vi "FL defuzzify output variables.vi"(7 "max num consequent membership fcns":i32, 9 "output membership factors (u)":dbl[][](array[numeric]), 11 "fuzzy system in":T1={"input variables"=[], "output variables"=[], "rules"=[], "defuzzification method"=0, "description"="\r\n", "user MF interpolating polynomials"=[]} {"user MF interpolating polynomials"."coa_x(y) coeff" format="%.4g"; "user MF interpolating polynomials"."Area(y) coeff" format="%.4g"; "user MF interpolating polynomials"."X(y) coeff" format="%.4g"; "user MF interpolating polynomials"."Y(x) coeff" format="%.4g"; "user MF interpolating polynomials"."Y" format="%.4g"; "user MF interpolating polynomials"."X" format="%.4g"; "defuzzification method" items=["Center of Area", "Modified Center of Area", "Center of Sums", "Center of Maximum", "Mean of Maximum"]; "rules"."consequents"."Var Index" min=0; "rules"."consequents"."Cond" items=["=", "!="]; "rules"."consequents"."MF Index" min=0; "rules"."antecedents"."Var Index" min=0; "rules"."antecedents"."Cond" items=["=", "!="]; "rules"."antecedents"."MF Index" min=0; "rules"."consequent implication" items=["Minimum", "Product"]; "rules"."antecedent connective" items=["AND (Minimum)", "AND (Product)", "OR (Maximum)", "OR (Probabilistic)"]; "output variables"."MFs"."shape" items=["Triangle", "Trapezoid", "Singleton", "Sigmoid", "Gaussian", "User-Defined"]; "input variables"."MFs"."shape" items=["Triangle", "Trapezoid", "Singleton", "Sigmoid", "Gaussian", "User-Defined"]}) -> (1 "output membership factors (u)":dbl[][](array[numeric]), 2 "output variables":dbl[](array[numeric])=[2.4048035734913955], 3 "fuzzy system out":T1 {"user MF interpolating polynomials"."coa_x(y) coeff" format="%.4g"; "user MF interpolating polynomials"."Area(y) coeff" format="%.4g"; "user MF interpolating polynomials"."X(y) coeff" format="%.4g"; "user MF interpolating polynomials"."Y(x) coeff" format="%.4g"; "user MF interpolating polynomials"."Y" format="%.4g"; "user MF interpolating polynomials"."X" format="%.4g"; "defuzzification method" items=["Center of Area", "Modified Center of Area", "Center of Sums", "Center of Maximum", "Mean of Maximum"]; "rules"."consequents"."Var Index" min=0; "rules"."consequents"."Cond" items=["=", "!="]; "rules"."consequents"."MF Index" min=0; "rules"."antecedents"."Var Index" min=0; "rules"."antecedents"."Cond" items=["=", "!="]; "rules"."antecedents"."MF Index" min=0; "rules"."consequent implication" items=["Minimum", "Product"]; "rules"."antecedent connective" items=["AND (Minimum)", "AND (Product)", "OR (Maximum)", "OR (Probabilistic)"]; "output variables"."MFs"."shape" items=["Triangle", "Trapezoid", "Singleton", "Sigmoid", "Gaussian", "User-Defined"]; "input variables"."MFs"."shape" items=["Triangle", "Trapezoid", "Singleton", "Sigmoid", "Gaussian", "User-Defined"]})   [LabVIEW 2020, in "NI_Fuzzy_Logic_API.lvlib"]
uses:
  <vilib>/addons/Fuzzy Logic/NI_Fuzzy_Logic_API.lvlib
  <vilib>/addons/Fuzzy Logic/TypeDefs/FL System.ctl
  <vilib>/addons/Fuzzy Logic/TypeDefs/FL Variable.ctl
  <vilib>/addons/Fuzzy Logic/TypeDefs/FL Membership Function.ctl
  <vilib>/addons/Fuzzy Logic/TypeDefs/FL Membership Function Shape.ctl
  <vilib>/addons/Fuzzy Logic/TypeDefs/FL Rule.ctl
  <vilib>/addons/Fuzzy Logic/TypeDefs/FL Antecedent.ctl
  <vilib>/addons/Fuzzy Logic/TypeDefs/FL Modifier.ctl
  <vilib>/addons/Fuzzy Logic/TypeDefs/FL Antecedent Connective.ctl
  <vilib>/addons/Fuzzy Logic/TypeDefs/FL Consequent.ctl
  <vilib>/addons/Fuzzy Logic/TypeDefs/FL Consequent Implication.ctl
  <vilib>/addons/Fuzzy Logic/TypeDefs/FL Defuzzification.ctl
  <vilib>/addons/Fuzzy Logic/TypeDefs/FL Interpolating polynomials.ctl
  <vilib>/Analysis/1siggen.llb/Ramp Pattern by Samples.vi
  <vilib>/Analysis/8numeric.llb/1D Numeric Integration.vi
  <vilib>/Analysis/NI_AALPro.lvlib
  <vilib>/Analysis/NI_AALBase.lvlib
panel:
  # "IF"
  # "THEN"
  # "IF"
  # "THEN"
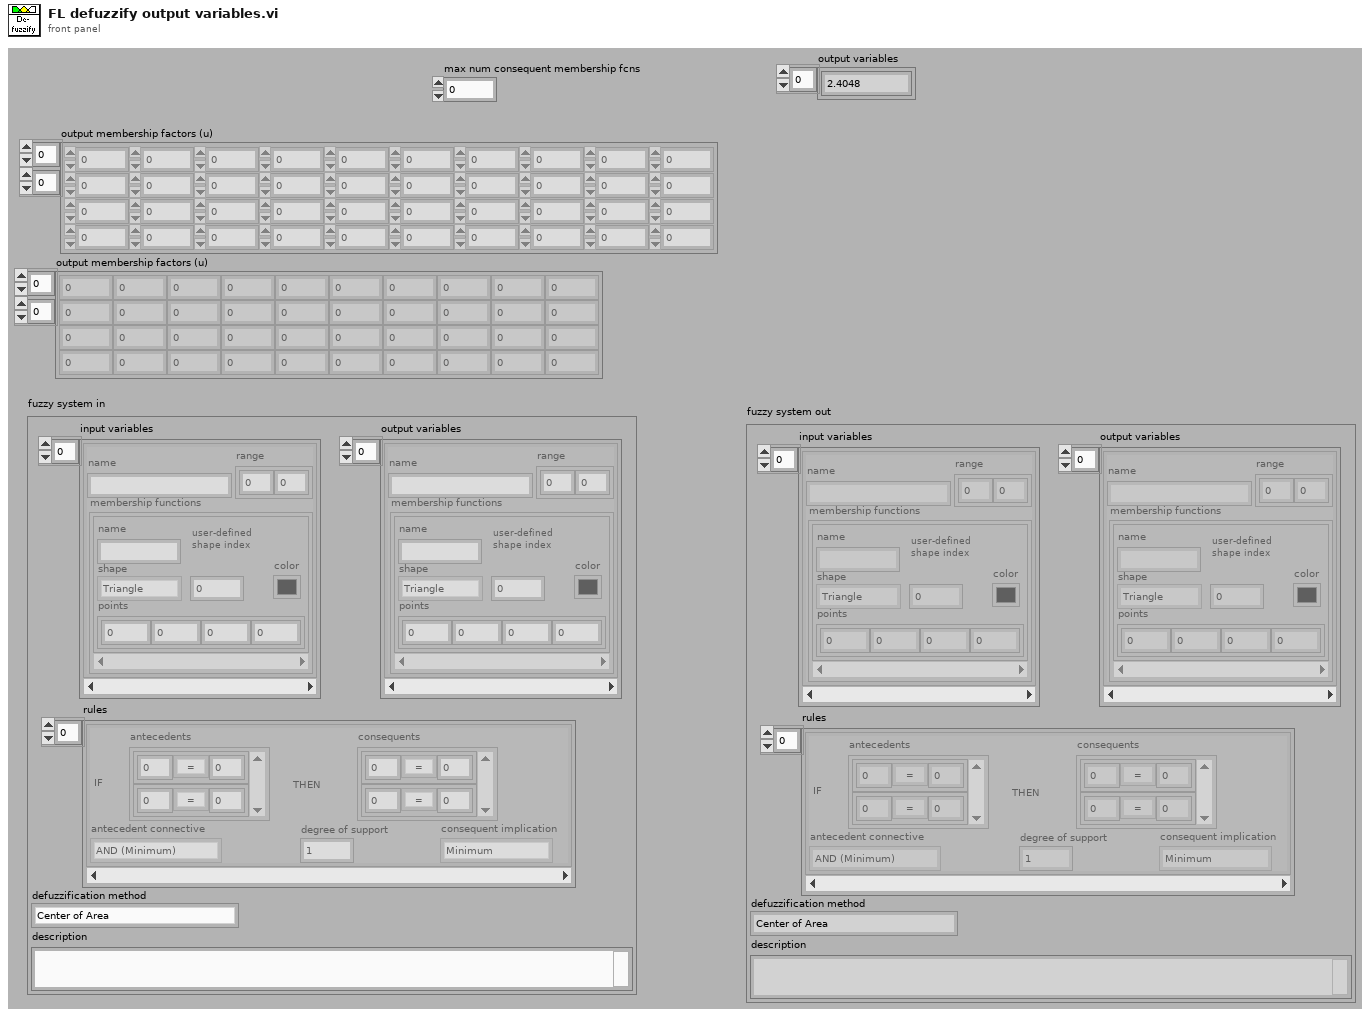
[diagram p1: front panel]
types:
  T1 = typedef "NI_Fuzzy_Logic_API.lvlib/FL System.ctl" = cluster{"input variables":T2[], "output variables":T2[], "rules":T5[], "defuzzification method":T11, "description":string, "user MF interpolating polynomials":T12[]}
  T2 = typedef "NI_Fuzzy_Logic_API.lvlib/FL Variable.ctl" = cluster{"name":string, "range":dbl[], "MFs":T3[]}
  T3 = typedef "NI_Fuzzy_Logic_API.lvlib/FL Membership Function.ctl" = cluster{"name":string, "shape":T4, "points":dbl[], "color":u32, "user-defined shape index":i32}
  T4 = typedef "NI_Fuzzy_Logic_API.lvlib/FL Membership Function Shape.ctl" = u16
  T5 = typedef "NI_Fuzzy_Logic_API.lvlib/FL Rule.ctl" = cluster{"antecedents":T6[], "antecedent connective":T8, "consequents":T9[], "consequent implication":T10, "degree of support":dbl}
  T6 = typedef "NI_Fuzzy_Logic_API.lvlib/FL Antecedent.ctl" = cluster{"Var Index":i32, "MF Index":i32, "Cond":T7}
  T7 = typedef "NI_Fuzzy_Logic_API.lvlib/FL Modifier.ctl" = u16
  T8 = typedef "NI_Fuzzy_Logic_API.lvlib/FL Antecedent Connective.ctl" = u16
  T9 = typedef "NI_Fuzzy_Logic_API.lvlib/FL Consequent.ctl" = cluster{"Var Index":i32, "MF Index":i32, "Cond":T7}
  T10 = typedef "NI_Fuzzy_Logic_API.lvlib/FL Consequent Implication.ctl" = u16
  T11 = typedef "NI_Fuzzy_Logic_API.lvlib/FL Defuzzification.ctl" = u16
  T12 = typedef "NI_Fuzzy_Logic_API.lvlib/FL Interpolating polynomials.ctl" = cluster{"X":dbl[], "Y":dbl[], "Y(x) coeff":dbl[][], "X(y) coeff":dbl[][], "Area(y) coeff":dbl[][], "coa_x(y) coeff":dbl[][]}
  T13 = enum32{"Trapezoidal Rule", "Simpson's Rule", "Simpson's 3/8 Rule", "Bode Rule"}
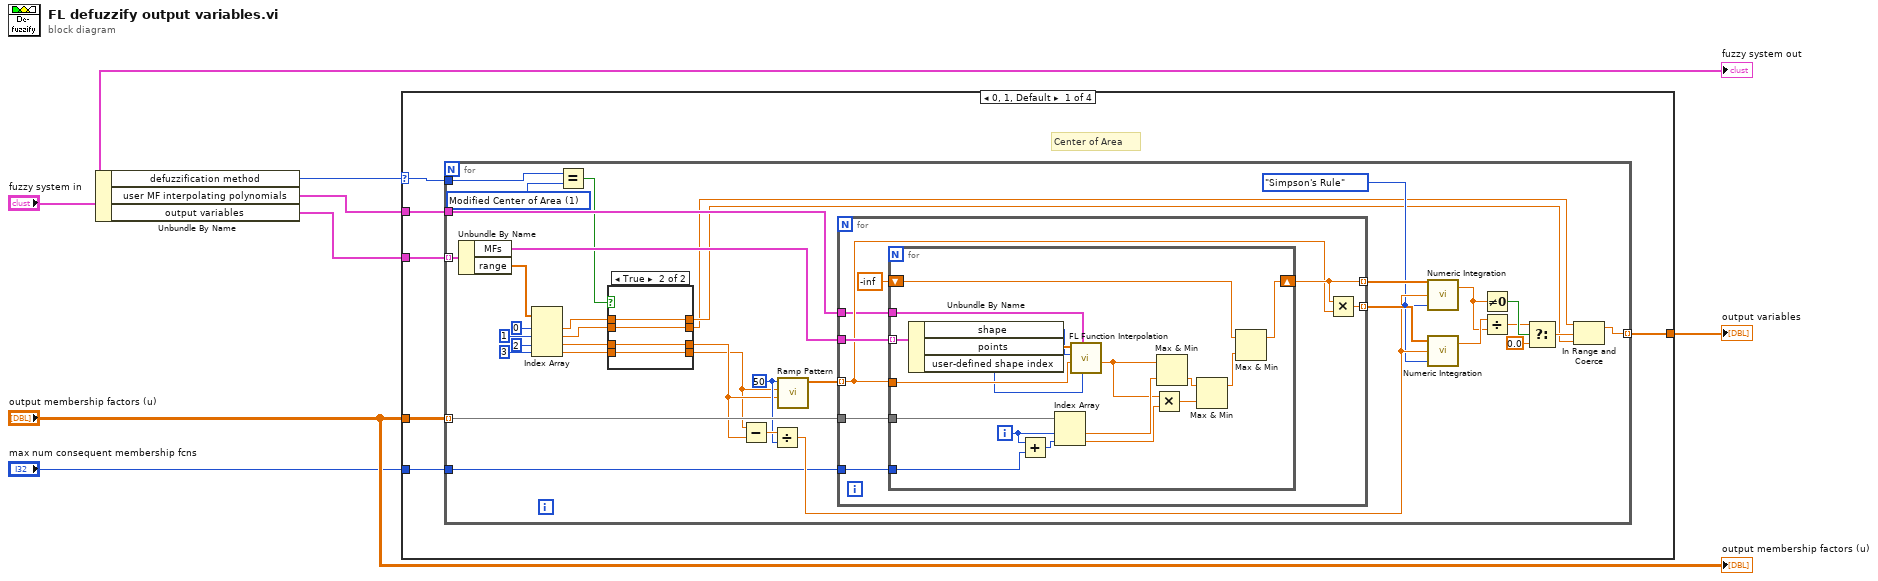
[diagram p0: block diagram]
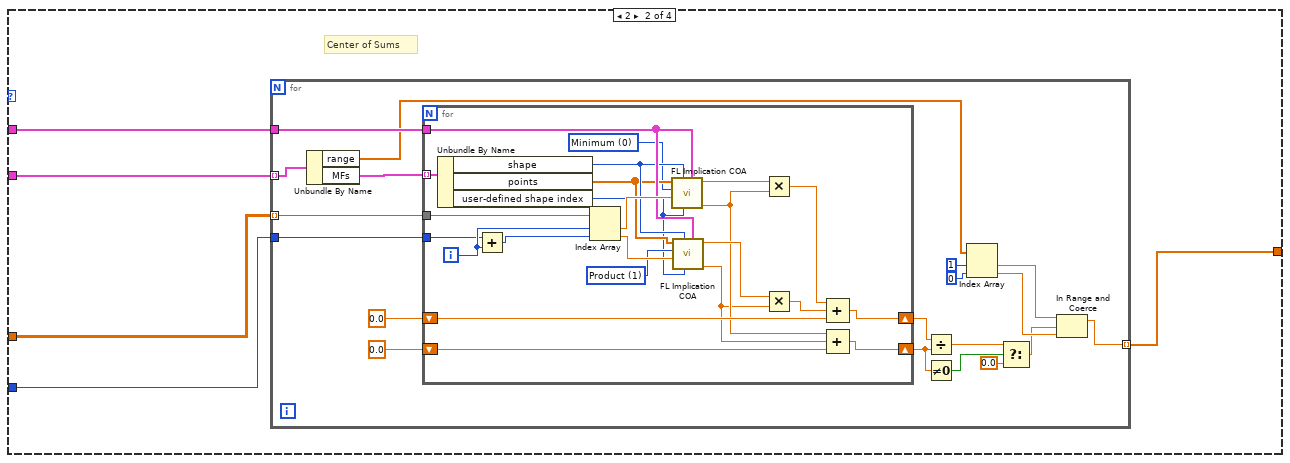
[diagram p3: hidden frame]
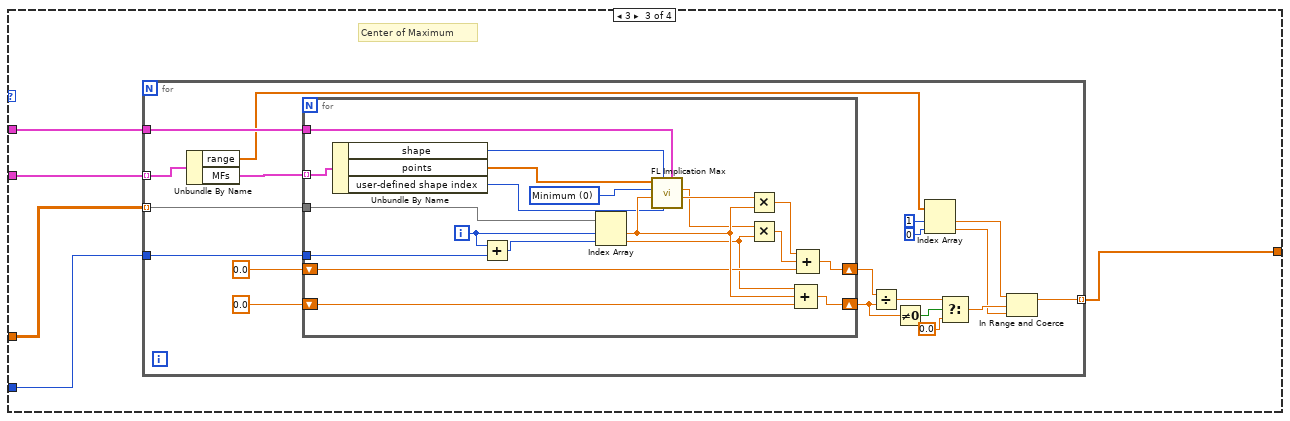
[diagram p4: hidden frame]
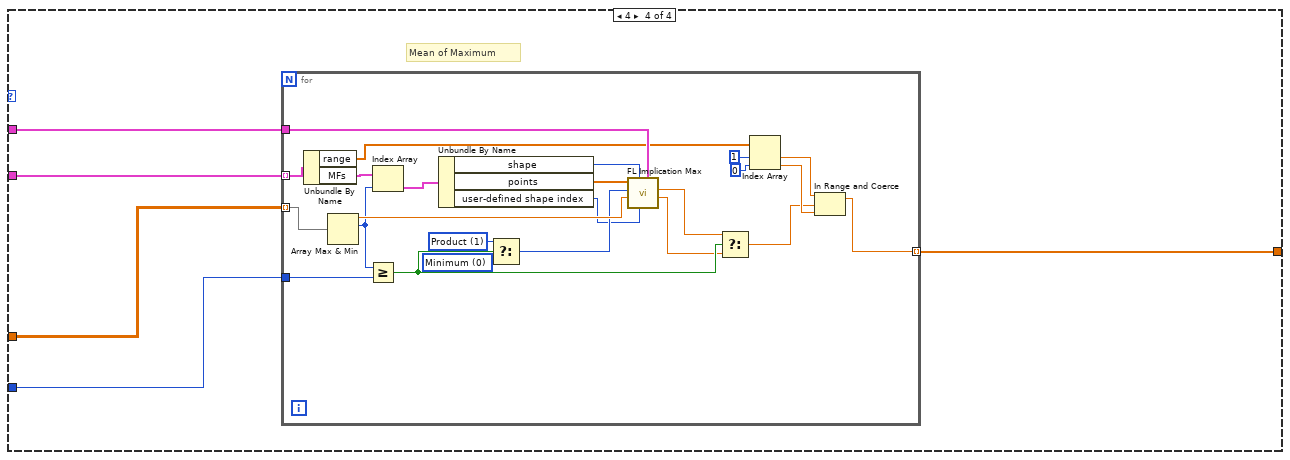
[diagram p5: hidden frame]
diagram:
  n1 = Unbundle By Name("fuzzy system in") -> ("defuzzification method"=w5:T11, "user MF interpolating polynomials"=w4:T12[], "output variables"=w3:T2[])
  n2 = case shown="0, 1, Default" w5 {
    selector: w5 -> [w8 _ _ _]
    tunnel: "output membership factors (u)" -> [w13 w85 w132 w176]
    tunnel: w3 -> [w12 w84 w131 w175]
    tunnel: [w11 w83 w129 w173] -> w7
    tunnel: w4 -> [w10 w82 w130 w174]
    tunnel: "max num consequent membership fcns" -> [w9 w81 w128 w172]
    frame 0, 1, Default {
      # "Center of Area"
      n3 = for {
        tunnel: w13 -> [w45] mode=indexing
        tunnel: w12 -> [w48] mode=indexing
        tunnel: [w29] -> w11 mode=indexing
        tunnel: w10 -> [w37]
        tunnel: w9 -> [w31]
        tunnel: w8 -> [w14]
        w26 = T11 1 items=["Center of Area", "Modified Center of Area", "Center of Sums", "Center of Maximum", "Mean of Maximum"] ("y")
        w38 = T13."Simpson's Rule" ("integration method")
        w42 = 50 ("samples")
        n4 = Unbundle By Name(w48) -> ("MFs"=w46:T3[], "range"=w47:dbl[])
        n5 = Index Array(array=w47, index #1=0 ("index"), index #2=1 ("index"), index #3=2 ("index"), index #4=3 ("index")) -> (element #1=w22:dbl, element #2=w21:dbl, element #3=w20:dbl, element #4=w19:dbl)
        n6 = Equal?(x=w14, y=w26) -> (x = y?=w23:bool)
        n7 = case shown="True" w23 {
          tunnel: w22 -> [w50 w54]
          tunnel: w21 -> [w49 w53]
          tunnel: w20 -> [_ w52]
          tunnel: w19 -> [_ w51]
          tunnel: [w50 w54] -> w17
          tunnel: [w49 w53] -> w16
          tunnel: [w50 w52] -> w18
          tunnel: [w49 w51] -> w15
          frame False {
          }
          frame True {
          }
        }
        n8 = Subtract(x=w15, y=w18) -> (x-y=w43:dbl)
        n9 = Divide(x=w43, y=w42) -> (x/y=w39:dbl)
        n10 = call-poly <vilib>:"Ramp Pattern.vi"("start"=w18, "end"=w15, "samples"=w42) -> ("Ramp Pattern"=w44:dbl[])  [unwired: 7 in, 1 out]
        n11 = for {
          tunnel: w46 -> [w61]
          tunnel: w45 -> [w60]
          tunnel: w44 -> [w58] mode=indexing
          tunnel: [w59] -> w41 mode=indexing
          tunnel: [w57] -> w40 mode=indexing
          tunnel: w37 -> [w56]
          tunnel: w31 -> [w55]
          n12 = for {
            tunnel: w61 -> [w79] mode=indexing
            tunnel: w60 -> [w80]
            shift-right: [w75] -> w59
            shift-left: -inf -> [w76]
            tunnel: w58 -> [w74]
            tunnel: w56 -> [w65]
            tunnel: w55 -> [w68]
            i -> [w69]
            n13 = Unbundle By Name(w79) -> ("shape"=w64:T4, "points"=w78:dbl[], "user-defined shape index"=w63:i32)
            n14 = Add(x=w69, y=w68) -> (x+y=w67:i32)
            n15 = Index Array(array=w80, index #1=w69, index #2=w67) -> (element #1=w77:dbl, element #2=w66:dbl)
            n16 = call <vilib>:"FL Function Interpolation.vi"("user-defined \nshape index"=w63, "user MF interpolating polynomials"=w65, "Input Data"=w74, "shape"=w64, "Points"=w78) -> ("Membership"=w73:dbl)  [unwired: 1 in, 5 out]
            n17 = Multiply(x=w73, y=w66) -> (x*y=w72:dbl)
            n18 = Max & Min(x=w73, y=w77) -> (min(x,y)=w71:dbl)  [unwired: 1 out]
            n19 = Max & Min(x=w71, y=w72) -> (max(x,y)=w70:dbl)  [unwired: 1 out]
            n20 = Max & Min(x=w76, y=w70) -> (max(x,y)=w75:dbl)  [unwired: 1 out]
          }
          n21 = Multiply(x=w59, y=w58) -> (x*y=w57:dbl)
        }
        n22 = call-poly <vilib>:"Numeric Integration.vi"("integration method"=w38, "dt"=w39, "Input Array"=w41) -> ("result"=w35:dbl)  [unwired: 1 out]
        n23 = call-poly <vilib>:"Numeric Integration.vi"("integration method"=w38, "dt"=w39, "Input Array"=w40) -> ("result"=w36:dbl)  [unwired: 1 out]
        n24 = Not Equal To 0?(x=w35) -> (x != 0?=w34:bool)
        n25 = Divide(x=w36, y=w35) -> (x/y=w33:dbl)
        n26 = Select(t=w33, s=w34, f=0.0) -> (s? t:f=w30:dbl)
        n27 = In Range and Coerce(upper limit=w16, x=w30, lower limit=w17) -> (coerced(x)=w29:dbl)  [unwired: 1 out]
      }
    }
    frame 2 {
      # "Center of Sums"
      n28 = for {
        tunnel: w85 -> [w104] mode=indexing
        tunnel: w84 -> [w103] mode=indexing
        tunnel: w82 -> [w101]
        tunnel: [w86] -> w83 mode=indexing
        tunnel: w81 -> [w93]
        n29 = Unbundle By Name(w103) -> ("range"=w92:dbl[], "MFs"=w102:T3[])
        n30 = for {
          tunnel: w104 -> [w121]
          tunnel: w102 -> [w127] mode=indexing
          tunnel: w101 -> [w115]
          shift-right: [w125] -> w98
          shift-left: 0.0 -> [w126]
          shift-right: [w123] -> w96
          shift-left: 0.0 -> [w124]
          tunnel: w93 -> [w118]
          i -> [w119]
          w106 = T10 0 items=["Minimum", "Product"] ("Implication")
          w107 = T10 1 items=["Minimum", "Product"] ("Implication")
          n31 = Unbundle By Name(w127) -> ("shape"=w114:T4, "points"=w113:dbl[], "user-defined shape index"=w105:i32)
          n32 = Add(x=w118, y=w119) -> (x+y=w120:i32)
          n33 = Index Array(array=w121, index #1=w119, index #2=w120) -> (element #1=w116:dbl, element #2=w117:dbl)
          n34 = call <vilib>:"FL Implication COA.vi"("user MF interpolating polynomials"=w115, "user-defined \nshape index"=w105, "Function"=w114, "Weight"=w116, "Implication"=w106, "Points (X)"=w113) -> ("area"=w109:dbl, "X(CoA)"=w122:dbl)  [unwired: 4 out]
          n35 = call <vilib>:"FL Implication COA.vi"("user MF interpolating polynomials"=w115, "user-defined \nshape index"=w105, "Function"=w114, "Weight"=w117, "Implication"=w107, "Points (X)"=w113) -> ("area"=w108:dbl, "X(CoA)"=w112:dbl)  [unwired: 4 out]
          n36 = Multiply(x=w122, y=w109) -> (x*y=w111:dbl)
          n37 = Multiply(x=w112, y=w108) -> (x*y=w110:dbl)
          n38 = Compound Arithmetic op=ADD(w111, w110, w126) -> (w125:dbl)
          n39 = Compound Arithmetic op=ADD(w109, w108, w124) -> (w123:dbl)
        }
        n40 = Divide(x=w98, y=w96) -> (x/y=w95:dbl)
        n41 = Not Equal To 0?(x=w96) -> (x != 0?=w97:bool)
        n42 = Index Array(array=w92, index #1=1 ("index"), index #2=0 ("index")) -> (element #1=w89:dbl, element #2=w88:dbl)
        n43 = Select(t=w95, s=w97, f=0.0) -> (s? t:f=w87:dbl)
        n44 = In Range and Coerce(upper limit=w89, x=w87, lower limit=w88) -> (coerced(x)=w86:dbl)  [unwired: 1 out]
      }
    }
    frame 3 {
      # "Center of Maximum"
      n45 = for {
        tunnel: w132 -> [w151] mode=indexing
        tunnel: w131 -> [w150] mode=indexing
        tunnel: w130 -> [w148]
        tunnel: [w135] -> w129 mode=indexing
        tunnel: w128 -> [w140]
        n46 = Unbundle By Name(w150) -> ("range"=w137:dbl[], "MFs"=w149:T3[])
        n47 = for {
          tunnel: w151 -> [w163]
          tunnel: w149 -> [w171] mode=indexing
          tunnel: w148 -> [w168]
          shift-right: [w166] -> w145
          shift-left: 0.0 -> [w161]
          shift-right: [w164] -> w142
          shift-left: 0.0 -> [w165]
          tunnel: w140 -> [w159]
          i -> [w160]
          w153 = T10 0 items=["Minimum", "Product"] ("Implication")
          n48 = Unbundle By Name(w171) -> ("shape"=w170:T4, "points"=w169:dbl[], "user-defined shape index"=w152:i32)
          n49 = Add(x=w160, y=w159) -> (x+y=w158:i32)
          n50 = Index Array(array=w163, index #1=w160, index #2=w158) -> (element #1=w162:dbl, element #2=w156:dbl)
          n51 = call <vilib>:"FL Implication Max.vi"("user MF interpolating polynomials"=w168, "user-defined \nshape index"=w152, "Function"=w170, "Weight"=w162, "Implication"=w153, "Points (X)"=w169) -> ("X(Max)"=w167:dbl, "X(Max) product"=w157:dbl)  [unwired: 4 out]
          n52 = Multiply(x=w167, y=w162) -> (x*y=w155:dbl)
          n53 = Multiply(x=w157, y=w156) -> (x*y=w154:dbl)
          n54 = Compound Arithmetic op=ADD(w156, w162, w165) -> (w164:dbl)
          n55 = Compound Arithmetic op=ADD(w155, w154, w161) -> (w166:dbl)
        }
        n56 = Divide(x=w145, y=w142) -> (x/y=w141:dbl)
        n57 = Not Equal To 0?(x=w142) -> (x != 0?=w144:bool)
        n58 = Index Array(array=w137, index #1=1 ("index"), index #2=0 ("index")) -> (element #1=w134:dbl, element #2=w133:dbl)
        n59 = Select(t=w141, s=w144, f=0.0) -> (s? t:f=w136:dbl)
        n60 = In Range and Coerce(upper limit=w134, x=w136, lower limit=w133) -> (coerced(x)=w135:dbl)  [unwired: 1 out]
      }
    }
    frame 4 {
      # "Mean of Maximum"
      n61 = for {
        tunnel: w176 -> [w198] mode=indexing
        tunnel: w175 -> [w200] mode=indexing
        tunnel: w174 -> [w199]
        tunnel: [w180] -> w173 mode=indexing
        tunnel: w172 -> [w191]
        w179 = T10 1 items=["Minimum", "Product"] ("Implication")
        w178 = T10 0 items=["Minimum", "Product"] ("Implication")
        n62 = Unbundle By Name(w200) -> ("range"=w186:dbl[], "MFs"=w194:T3[])
        n63 = Array Max & Min(array=w198) -> (max value=w195:dbl, max index (indices)=w192:i32)  [unwired: 2 out]
        n64 = Greater Or Equal?(x=w192, y=w191) -> (x >= y?=w190:bool)
        n65 = Index Array(array=w194, index=w192) -> (element=w193:T3)
        n66 = Unbundle By Name(w193) -> ("shape"=w197:T4, "points"=w196:dbl[], "user-defined shape index"=w177:i32)
        n67 = Select(t=w179, s=w190, f=w178) -> (s? t:f=w189:T10)
        n68 = call <vilib>:"FL Implication Max.vi"("user MF interpolating polynomials"=w199, "user-defined \nshape index"=w177, "Function"=w197, "Weight"=w195, "Implication"=w189, "Points (X)"=w196) -> ("X(Max)"=w187:dbl, "X(Max) product"=w188:dbl)  [unwired: 4 out]
        n69 = Select(t=w188, s=w190, f=w187) -> (s? t:f=w181:dbl)
        n70 = Index Array(array=w186, index #1=1 ("index"), index #2=0 ("index")) -> (element #1=w183:dbl, element #2=w182:dbl)
        n71 = In Range and Coerce(upper limit=w183, x=w181, lower limit=w182) -> (coerced(x)=w180:dbl)  [unwired: 1 out]
      }
    }
  }
  "output variables" <- w7
  "output membership factors (u)" <- "output membership factors (u)"
  "fuzzy system out" <- "fuzzy system in"
